vi "ConfigureStandardWaveform.vi"(8 "error in (no error)":errorcluster, 11 "FunctionGenerator in":refnum<class "FunctionGenerator.lvclass">) -> (0 "error out":errorcluster, 3 "FunctionGenerator out":refnum<class "FunctionGenerator.lvclass">)   [LabVIEW 2020, in "FunctionGenerator.lvclass"]
uses:
  FunctionGenerator.lvclass
  C:/Code Projects/CircuitExplorer/AnalogDiscoveryFunction/AnalogDiscoveryFunction.lvclass
  FunctionGenerator.lvclass/FunctionGenerator.ctl
  OutputWaveform/OutputWaveform.lvclass/OutputWaveform.ctl
  AnalogDiscoveryFunction/AnalogDiscoveryFunction.lvclass/AnalogDiscoveryFunction.ctl
  OutputWaveform/GetWaveformParameters.vi
  AnalogDiscoveryFunction/GetInstrumentHandle.vi
  <vilib>/DigilentWF/DigilentWF.lvlib
  OutputWaveform/OutputWaveform.lvclass
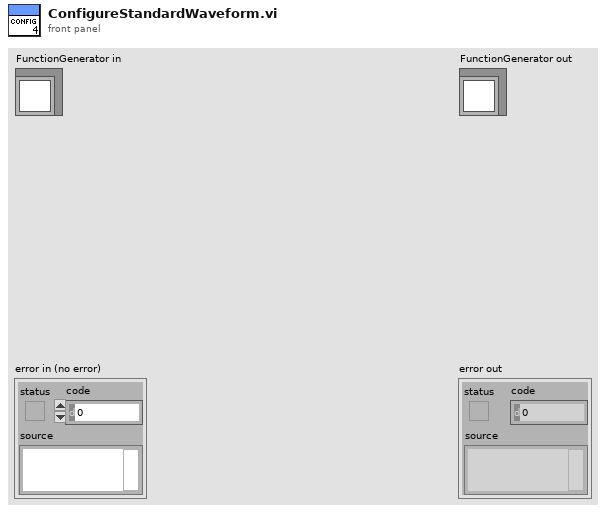
[diagram p1: front panel]
types:
  T1 = cluster{"Duty Cycle":dbl, "Frequency":dbl, "Waveform Function":i32, "Amplitude":dbl, "DC Offset":dbl}
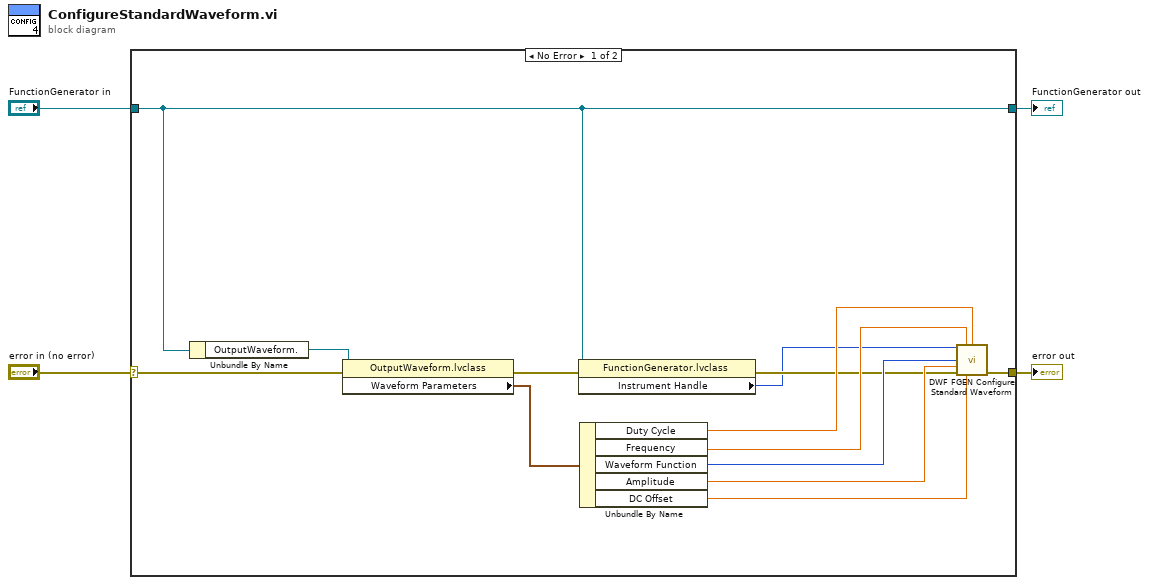
[diagram p0: block diagram]
diagram:
  n1 = case shown="No Error" "error in (no error)" {
    selector: "error in (no error)" -> [w16 w19]
    tunnel: [w17 w19] -> w3
    tunnel: [w8 w18] -> w1
    tunnel: "FunctionGenerator in" -> [w8 w18]
    frame No Error {
      n2 = Unbundle By Name(w8) -> ("OutputWaveform."=w15:refnum<class "OutputWaveform.lvclass">)
      n3 = property class="OutputWaveform.lvclass"(reference=w15, error in=w16) -> (error out=w7:errorcluster, "Waveform Parameters"=w14:T1)  [unwired: 1 out]
      n4 = property class="FunctionGenerator.lvclass"(reference=w8, error in=w7) -> (error out=w6:errorcluster, "Instrument Handle"=w5:u32)  [unwired: 1 out]
      n5 = Unbundle By Name(w14) -> ("Duty Cycle"=w9:dbl, "Frequency"=w10:dbl, "Waveform Function"=w11:i32, "Amplitude"=w12:dbl, "DC Offset"=w13:dbl)
      n6 = call <vilib>:"DWF FGEN Configure Standard Waveform.vi"("Instrument Handle In"=w5, "Frequency"=w10, "Duty Cycle"=w9, "Waveform Function"=w11, "Amplitude"=w12, "Error In"=w6, "DC Offset"=w13) -> ("Error Out"=w17:errorcluster)  [unwired: 7 in, 1 out]
    }
    frame Error {
    }
  }
  "error out" <- w3
  "FunctionGenerator out" <- w1
